vi "Escape XML Text.vi"(1 "String":string) -> (0 "Escaped":string)   [LabVIEW 2023, in "VILab.lvlib"]
uses:
  VILab.lvlib
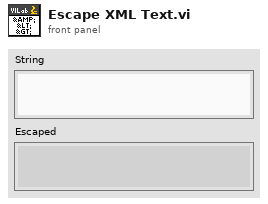
[diagram p1: front panel]
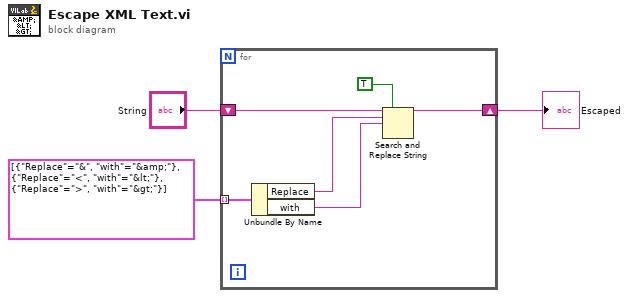
[diagram p0: block diagram]
diagram:
  n1 = for {
    tunnel: cluster{"Replace":string, "with":string}[] [{"Replace"="&", "with"="&amp;"}, {"Replace"="<", "with"="&lt;"}, {"Replace"=">", "with"="&gt;"}] -> [w8] mode=indexing
    shift-right: [w5] -> w1
    shift-left: "String" -> [w9]
    n2 = Unbundle By Name(w8) -> ("Replace"=w7:string, "with"=w6:string)
    n3 = Search and Replace String(replace all?=TRUE ("replace all? (F)"), input string=w9, search string=w7, replace string=w6) -> (result string=w5:string)  [unwired: 4 in, 3 out]
  }
  "Escaped" <- w1
